vi "Write Model2ICDASColumns.vi"(8 "error in (no error)":errorcluster, 10 "Model2ICDASColumns":string[](array[string]), 11 "AcPwrSimBase in":refnum<class "AcPwrSimBase.lvclass">) -> (0 "error out":errorcluster, 3 "AcPwrSimBase out":refnum<class "AcPwrSimBase.lvclass">)   [LabVIEW 2018, in "AcPwrPlugins.lvlib" / "AcPwrSimBase.lvclass"]
uses:
  AcPwrSimBase.lvclass
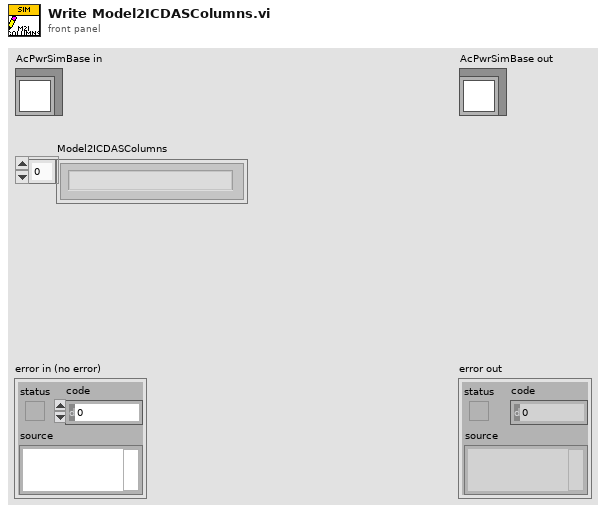
[diagram p1: front panel]
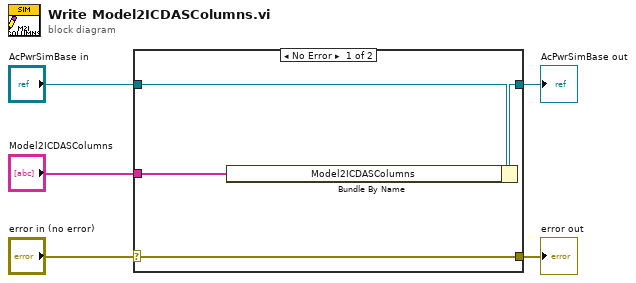
[diagram p0: block diagram]
diagram:
  n1 = case shown="No Error" "error in (no error)" {
    selector: "error in (no error)" -> [w9 w10]
    tunnel: [w9 w10] -> w4
    tunnel: [w7 w11] -> w2
    tunnel: "AcPwrSimBase in" -> [w8 w11]
    tunnel: "Model2ICDASColumns" -> [w6 _]
    frame No Error {
      n2 = Bundle By Name(cluster=w8, "Model2ICDASColumns"=w6) -> (w7:refnum<class "AcPwrSimBase.lvclass">)
    }
    frame Error {
    }
  }
  "error out" <- w4
  "AcPwrSimBase out" <- w2
